vi "PI Get List of Prompt Inputs.vi"(8 "error in (no error)":errorcluster, 11 "Connection Refnum In":T2) -> (0 "error out":errorcluster, 2 "Prompted Measurements":T1[](array[typedef]), 3 "Connection Refnum Out":T2)   [LabVIEW 2011]
uses:
  TypeDefs/PI Single Prompt Parameters.ctl
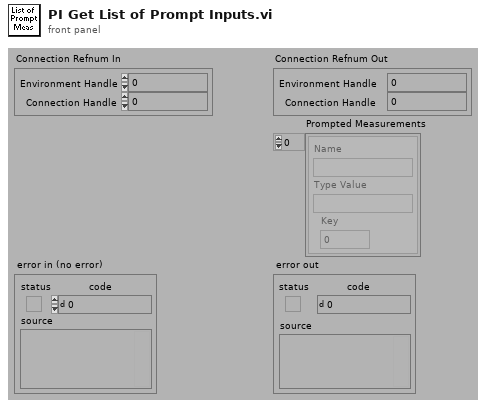
[diagram p1: front panel]
types:
  T1 = typedef "PI Single Prompt Parameters.ctl" = cluster{"Name":string, "Type Value":string, "Key":i32}
  T2 = cluster{"Environment Handle":i32, "Connection Handle":i32}
  T3 = typedef "Field Record.ctl" = cluster{"Key":i32, "Sequence ID":string, "Field ID":string, "Display Name":string, "Field Value":string, "Properties":T4, "Order":i32}
  T4 = typedef "Field Properties.ctl" = cluster{"Options":cluster{"System":bool, "System Value":bool, "Required":bool, "Set At Test":bool, "Measurement":bool}, "Next Item":T5}
  T5 = typedef "Field Next Item.ctl" = enum32{"Reset", "Retain", "Auto Inc."}
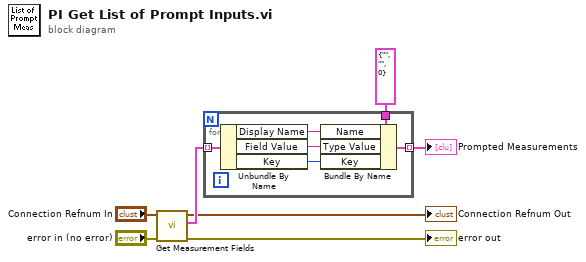
[diagram p0: block diagram]
diagram:
  n1 = call "Get Measurement Fields.vi"("error in (no error)"="error in (no error)", "Connection Refnum In"="Connection Refnum In") -> ("error out"=→"error out":errorcluster, "Measurement Field Array Out"=w4:T3[], "Connection Refnum Out"=→"Connection Refnum Out":T2)  [unwired: 6 in, 1 out]
  n2 = for {
    tunnel: w4 -> [w13] mode=indexing
    tunnel: T1 {"Name"="", "Type Value"="", "Key"=0} ("Prompt Parameters") -> [w12]
    tunnel: [w10] -> w2 mode=indexing
    n3 = Unbundle By Name(w13) -> ("Display Name"=w11:string, "Field Value"=w9:string, "Key"=w8:i32)
    n4 = Bundle By Name(cluster=w12, "Name"=w11, "Type Value"=w9, "Key"=w8) -> (w10:T1)
  }
  "Prompted Measurements" <- w2
